vi "isReporting.vi"(8 "error in (no error)":errorcluster, 11 "strict-JUnit in":refnum<class "strict-JUnit.lvclass">) -> (0 "error out":errorcluster, 2 "Exporting?":bool, 3 "strict-JUnit out":refnum<class "strict-JUnit.lvclass">)   [LabVIEW 2013, in "strict-JUnit.lvclass"]
uses:
  strict-JUnit.lvclass
  <vilib>/addons/_JKI Toolkits/Caraya/classes/Test Report.JUnit/Test Report.JUnit.lvclass
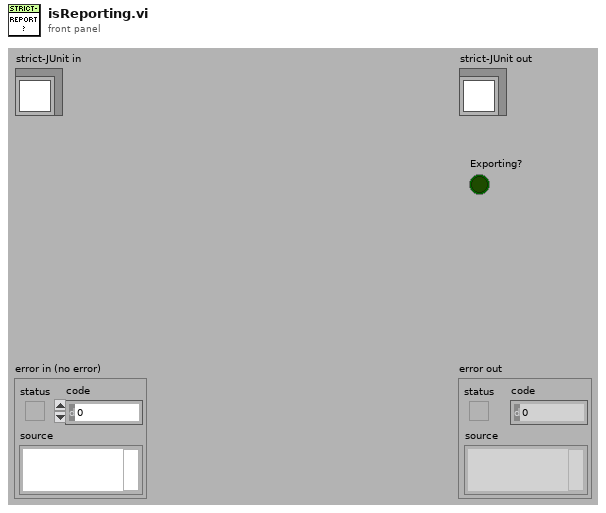
[diagram p1: front panel]
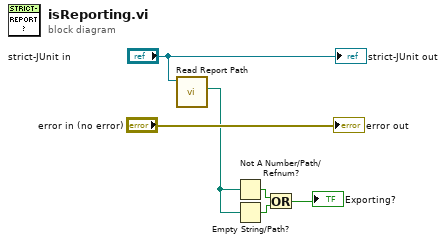
[diagram p0: block diagram]
diagram:
  n1 = call <vilib>:"Read Report Path.vi"("Test Report.JUnit in"="strict-JUnit in") -> ("Report Path"=w1:path)  [unwired: 9 in, 1 out]
  n2 = Not A Number/Path/Refnum?(number/path/refnum=w1) -> (NaN/Path/Refnum?=w5:bool)
  n3 = Empty String/Path?(string/path=w1) -> (empty?=w6:bool)
  n4 = Or(x=w5, y=w6) -> (x .or. y?=→"Exporting?":bool)
  "error out" <- "error in (no error)"
  "strict-JUnit out" <- "strict-JUnit in"
